vi "example multisequence.vi"() -> ()   [LabVIEW 2013]
uses:
  result/result.lvclass
  standard action/wait action/wait action.lvclass
  dispatcher/pool sizes.ctl
  result/result.lvclass/result.ctl
  result/get data.vi
  result/get error.vi
  result/get generating action.vi
  result/get owning task.vi
  result/get subresults.vi
  dispatcher/thread pool.lvclass
  standard reporters/event reporter/event reporter.lvclass
  standard tasks/sequence task/sequence task.lvclass
panel:
  out "times":u32[](array[numeric])
  out "owning task":string
  out "generating action":string
  out "error":errorcluster
  out "data":variant
  out "accessors:subresults":refnum<class "result.lvclass">[][](array[class])
  out "Array 4":string[](array[string])
  out "Array 3":string[](array[string])
  out "Array 2":errorcluster[](array[cluster])
  out "Array":variant[](array[variant])
  out "Time":u32
  out "result":refnum<class "result.lvclass">
  out "error out":errorcluster
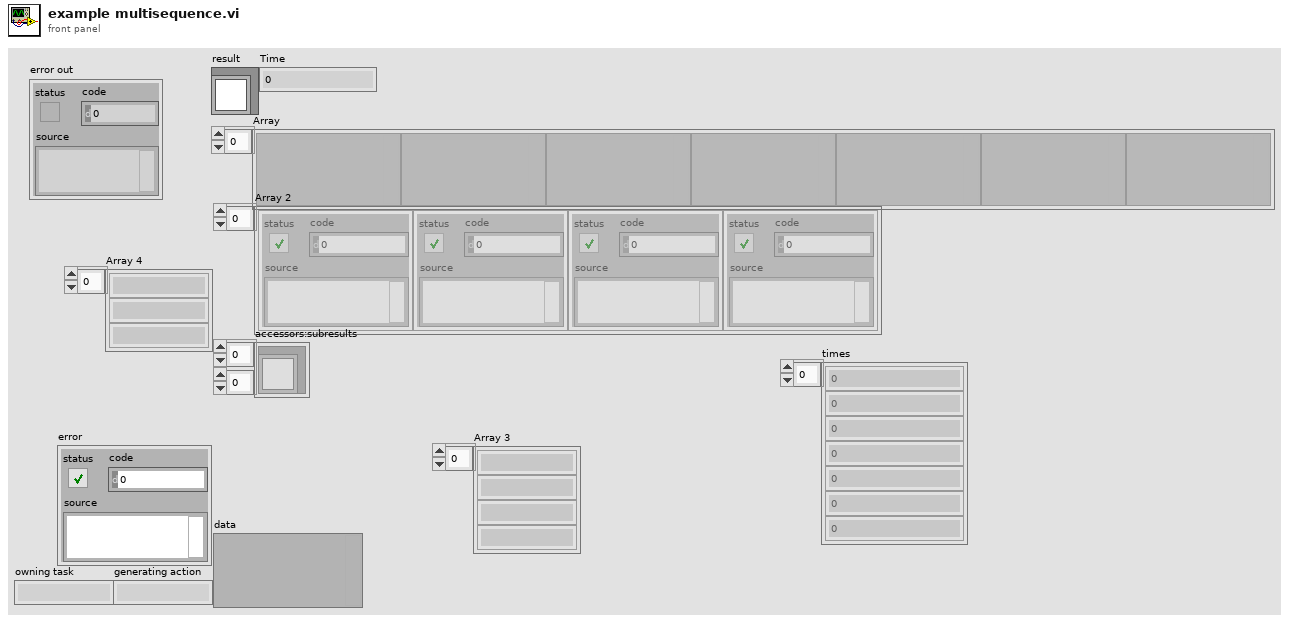
[diagram p1: front panel]
types:
  T1 = typedef "thread pool.lvclass/pool sizes.ctl" = cluster{"UI thread":u8, "standard":u8, "instrument I/O":u8, "data acquisition":u8, "other 1":u8, "other 2":u8}
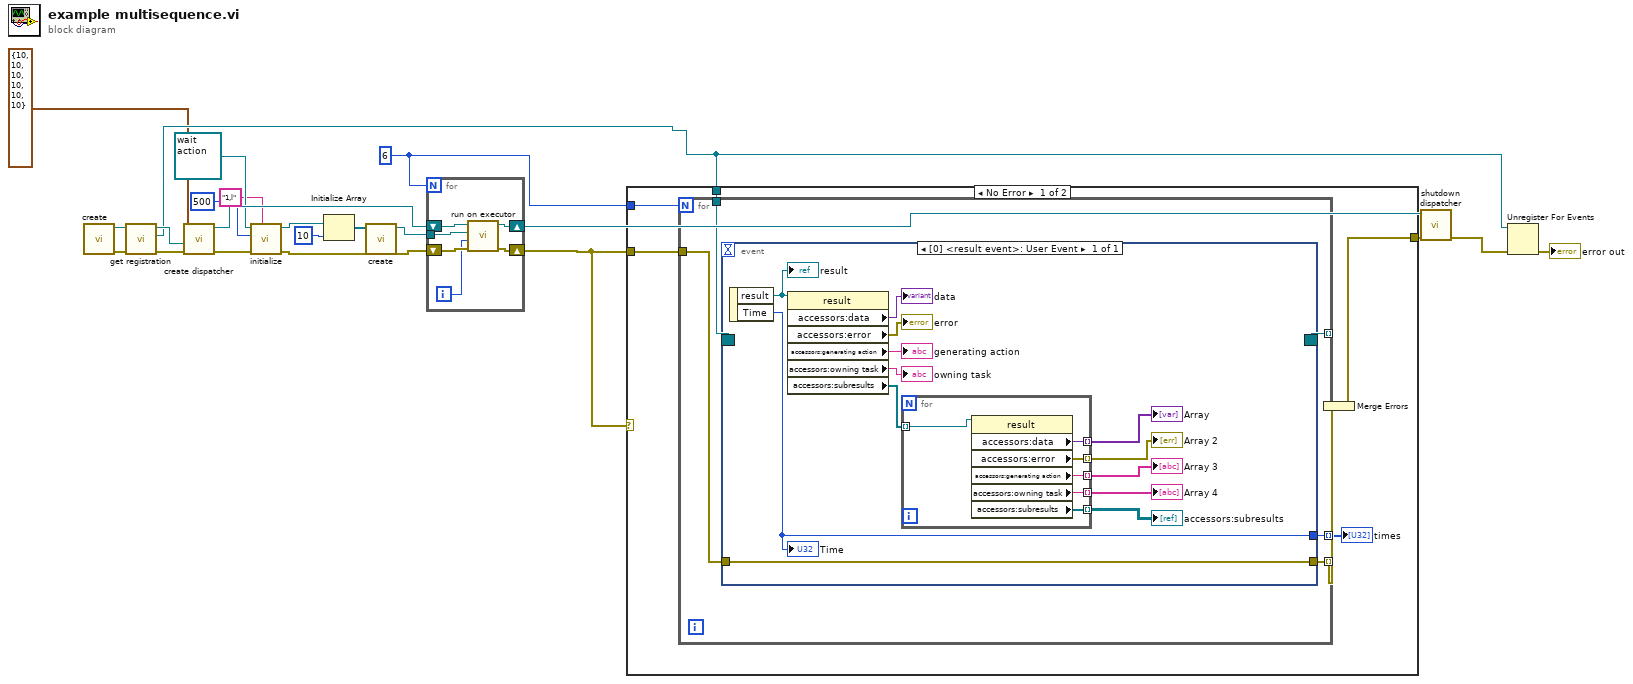
[diagram p0: block diagram]
diagram:
  w3 = 6
  n1 = call "create.vi"() -> ("error out"=w17:errorcluster, "event reporter out"=w18:refnum<class "event reporter.lvclass">)  [unwired: 10 in]
  n2 = call "get registration.vi"("error in"=w17, "event reporter in"=w18) -> ("error out"=w15:errorcluster, "result registration"=w4:refnum<event-registration>, "event reporter out"=w16:refnum<class "event reporter.lvclass">)  [unwired: 7 in]
  n3 = call "create dispatcher.vi"("error in"=w15, "default reporter"=w16, "initial pool sizes"=T1 {"UI thread"=10, "standard"=10, "instrument I/O"=10, "data acquisition"=10, "other 1"=10, "other 2"=10}) -> ("error out"=w20:errorcluster, "dispatcher"=w22:refnum<data-value>)  [unwired: 7 in]
  n4 = call-dynamic "initialize.vi"("action name"="1,l", "error in"=w20, "parameters"=500, "action in"=refnum<class "wait action.lvclass"> refnum ("wait action.lvclass")) -> ("error out"=w7:errorcluster, "action out"=w11:refnum<class "wait action.lvclass">)  [unwired: 6 in]
  n5 = Initialize Array(w11, 10 ("dimension size")) -> (w9:refnum<class "wait action.lvclass">[])
  n6 = call "create.vi"("actions"=w9) -> ("sequence task out"=w8:refnum<class "sequence task.lvclass">)  [unwired: 10 in]
  n7 = for {
    N: w3 -> [_]
    tunnel: w8 -> [w25]
    shift-right: [w27] -> w14
    shift-left: w22 -> [w28]
    shift-right: [w26] -> w2
    shift-left: w7 -> [w24]
    i -> [w23]
    n8 = call "run on executor.vi"("error in"=w24, "execution system"=w23, "task"=w25, "dispatcher"=w28) -> ("error out"=w26:errorcluster, "dispatcher out"=w27:refnum<data-value>)  [unwired: 6 in]
  }
  n9 = case shown="No Error" w2 {
    tunnel: w2 -> [w34 w59]
    tunnel: [w32 w59] -> w5
    tunnel: w4 -> [w31 _]
    tunnel: w3 -> [w30 _]
    frame No Error {
      n10 = for {
        N: w30 -> [_]
        tunnel: w31 -> [w39]
        tunnel: [w38] -> _ mode=indexing
        tunnel: [w37] -> w33 mode=indexing
        tunnel: w34 -> [w36]
        tunnel: [w35] -> w29 mode=indexing
        n11 = event shown="[0] <result event>: User Event" {
          selector: w39 -> [_]
          dyn-events: [_] -> w38
          timeout: _ -> [_]
          tunnel: [w52] -> w37
          tunnel: w36 -> [w52]
          tunnel: [w40] -> w35
          event User Event {
            n12 = event-data() -> ("result"=w51:refnum<class "result.lvclass">, "Time"=w40:u32)  [unwired: 1 in]
            "result" <- w51
            "Time" <- w40
            n13 = property class="result"(reference=w51) -> ("accessors:data"=→"data":variant, "accessors:error"=→"error":errorcluster, "accessors:generating action"=→"generating action":string, "accessors:owning task"=→"owning task":string, "accessors:subresults"=w50:refnum<class "result.lvclass">[])  [unwired: 1 in, 2 out]
            n14 = for {
              tunnel: w50 -> [w58] mode=indexing
              tunnel: [w57] -> w49 mode=indexing
              tunnel: [w56] -> w48 mode=indexing
              tunnel: [w55] -> w47 mode=indexing
              tunnel: [w54] -> w46 mode=indexing
              tunnel: [w53] -> w45 mode=indexing
              n15 = property class="result"(reference=w58) -> ("accessors:data"=w57:variant, "accessors:error"=w56:errorcluster, "accessors:generating action"=w55:string, "accessors:owning task"=w54:string, "accessors:subresults"=w53:refnum<class "result.lvclass">[])  [unwired: 1 in, 2 out]
            }
            "Array" <- w49
            "Array 2" <- w48
            "Array 3" <- w47
            "Array 4" <- w46
            "accessors:subresults" <- w45
          }
        }
      }
      "times" <- w29
      n16 = Merge Errors(w33) -> (w32:errorcluster)
    }
    frame Error {
    }
  }
  n17 = call "shutdown dispatcher.vi"("error in"=w5, "dispatcher"=w14) -> ("error out"=w13:errorcluster)  [unwired: 9 in]
  n18 = Unregister For Events(event registration refnum=w4, error in=w13) -> (error out=→"error out":errorcluster)
